vi "Battery Match.vi"(6 "ES ON Array In":bool[](array[boolean])=[FALSE, FALSE, FALSE, FALSE, FALSE, FALSE, FALSE, FALSE, FALSE, FALSE], 7 "Init":bool, 8 "Error In":errorcluster, 9 "PC Data":T2 {"Alarms 2" format="%016b"; "Faults 2" format="%016b"; "Alarms 1" format="%016b"; "Faults 1" format="%016b"; "Contactor FB" format="%.0b"; "DC Voltage SP" format="%2.1f"; "Clear Faults SP" format="%.0b"; "Neutral Current" format="%2.1f"; "AC Current - L2" format="%2.1f"; "AC Voltage - L2" format="%2.1f"; "Temperature" format="%2.1f"; "DC Voltage" format="%2.1f"; "AC Current SP" format="%2.1f"; "AC Voltage SP" format="%2.1f"; "Frequency SP" format="%2.1f"; "AC Frequency" format="%2.1f"; "AC Current - L1" format="%2.1f"; "AC Voltage- L1" format="%2.1f"}, 10 "ES System Data":T4={"Voltage"=0.0, "Current"=0.0, "SOC Avg"=0.0, "Faults"=0, "Alarms"=0, "# Strings"=0, "Max Temp"=0, "Min Temp"=0, "Max Cell Voltage"=0.0, "Min Cell Voltage"=0.0, "Energy Capacity"=0.0, "Energy Remaining"=0.0, "SOC Min"=0.0, "SOC Max"=0.0, "ES Fault"=FALSE, "String Select"=enum."3 Strings", "ES Com Fault"=FALSE, "SOH Avg"=0.0}, 11 "ES String Data":T6) -> (0 "Error Out":errorcluster, 1 "Matching Complete":bool=TRUE, 2 "ES ON Array Out":bool[](array[boolean]), 3 "Precharge Current Out":sgl)   [LabVIEW 2014]
uses:
  Controls/ES String Array.ctl
  Controls/ES String Data.ctl
  Controls/ES System Data.ctl
  Controls/StringSelector.ctl
  Controls/PC Data.ctl
  Controls/MicroZed Config Op Mode.ctl
  Controls/Battery Match State.ctl
panel:
  out "Last State":T1
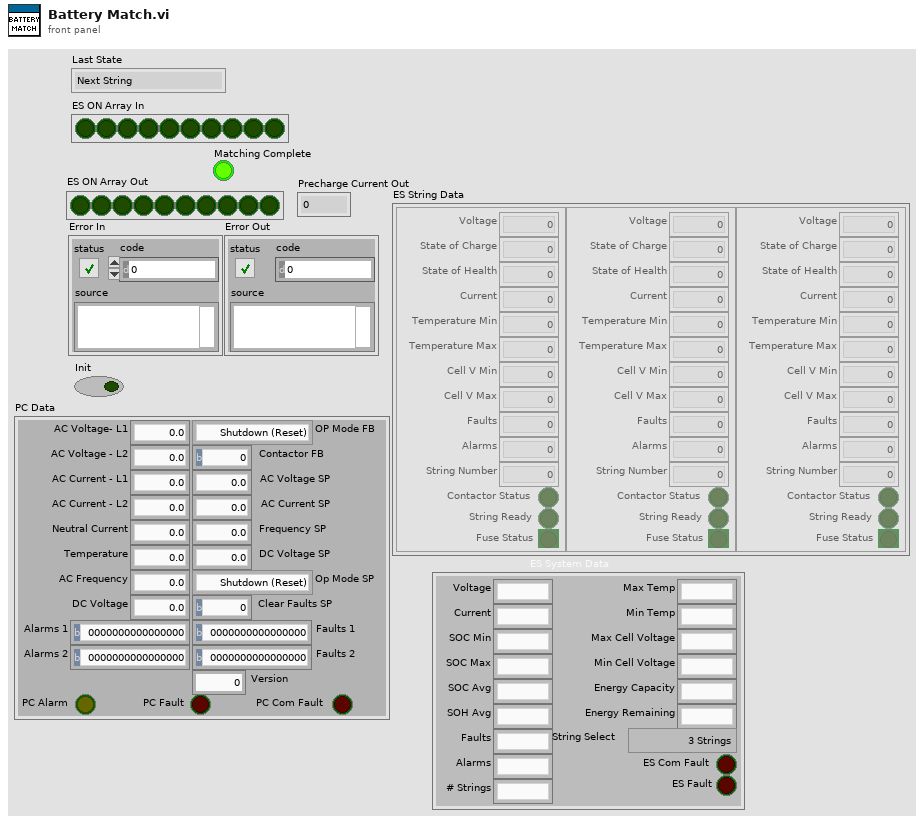
[diagram p1: front panel]
types:
  T1 = typedef "Battery Match State.ctl" = enum16{"Next String", "Charge String", "Matching Complete"}
  T2 = typedef "PC Data.ctl" = cluster{"AC Voltage- L1":dbl, "AC Voltage - L2":dbl, "AC Current - L1":dbl, "AC Current - L2":dbl, "Neutral Current":dbl, "Temperature":dbl, "AC Frequency":dbl, "DC Voltage":dbl, "AC Voltage SP":dbl, "AC Current SP":dbl, "Frequency SP":dbl, "Op Mode SP":T3, "Clear Faults SP":u16, "PC Com Fault":bool, "PC Fault":bool, "DC Voltage SP":dbl, "OP Mode FB":T3, "Contactor FB":u16, "Faults 1":u16, "Alarms 1":u16, "Faults 2":u16, "Alarms 2":u16, "PC Alarm":bool, "Version":u16}
  T3 = typedef "MicroZed Config Op Mode.ctl" = enum16{"Shutdown (Reset)", "Startup", "Idle", "Voltage Mode", "Current Mode", "Fault", "OL Voltage (Debug)", "No Data"}
  T4 = typedef "ES System Data.ctl" = cluster{"Voltage":sgl, "Current":sgl, "SOC Avg":sgl, "Faults":u16, "Alarms":u16, "# Strings":u16, "Max Temp":i16, "Min Temp":i16, "Max Cell Voltage":sgl, "Min Cell Voltage":sgl, "Energy Capacity":sgl, "Energy Remaining":sgl, "SOC Min":sgl, "SOC Max":sgl, "ES Fault":bool, "String Select":T5, "ES Com Fault":bool, "SOH Avg":sgl}
  T5 = typedef "StringSelector.ctl" = enum16{"1 String (1)", "1 String (2)", "1 String (3)", "2 Strings (1 2)", "2 Strings (2 3)", "2 Strings (1 3)", "3 Strings"}
  T6 = typedef "ES String Array.ctl" = T7[]
  T7 = typedef "ES String Data.ctl" = cluster{"Voltage":sgl, "State of Charge":sgl, "Current":sgl, "Temperature Min":i16, "Temperature Max":i16, "Faults":u16, "Alarms":u16, "String Number":u16, "Contactor Status":bool, "String Ready":bool, "Fuse Status":bool, "Cell V Max":dbl, "Cell V Min":dbl, "State of Health":sgl}
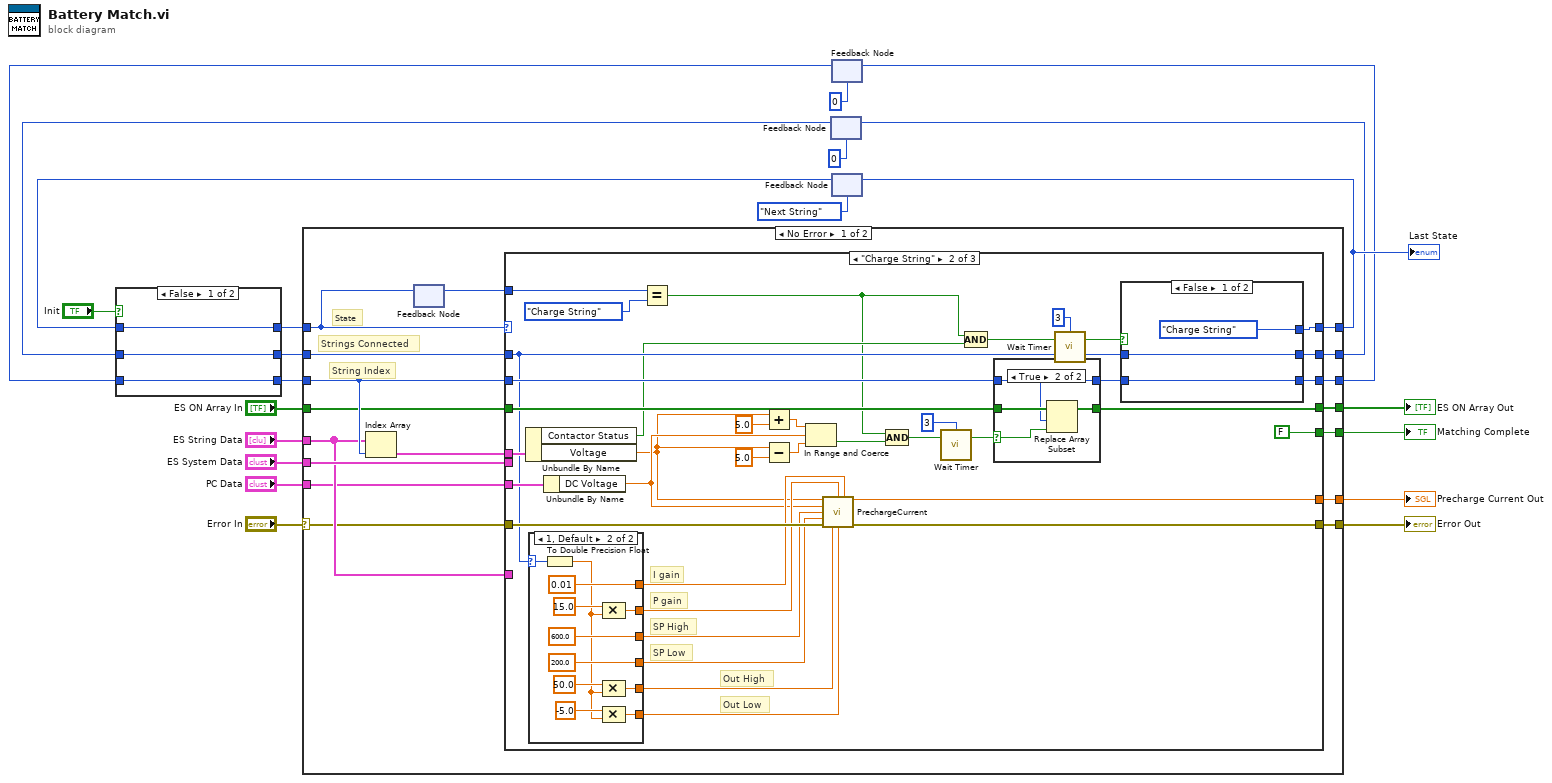
[diagram p0: block diagram]
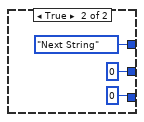
[diagram p2: hidden frame]
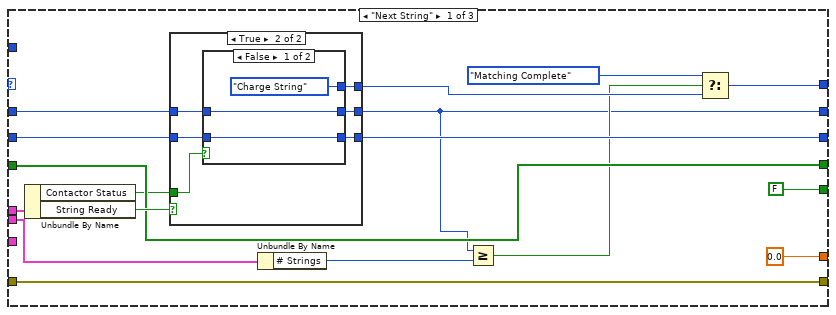
[diagram p3: hidden frame]
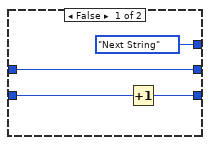
[diagram p4: hidden frame]
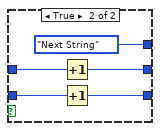
[diagram p5: hidden frame]
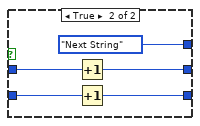
[diagram p6: hidden frame]
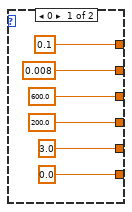
[diagram p8: hidden frame]
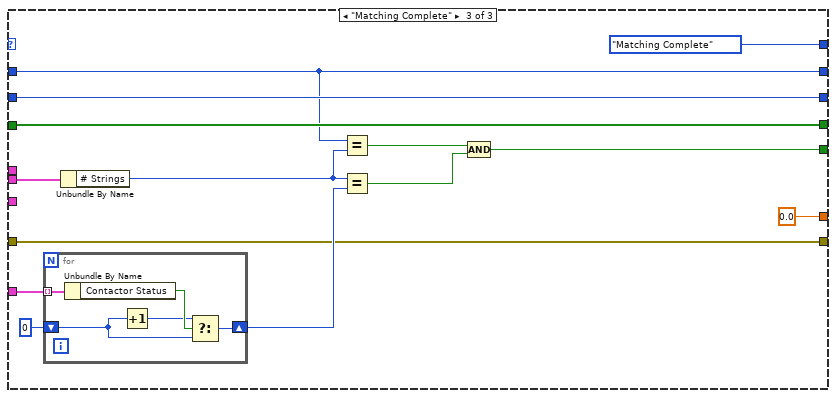
[diagram p9: hidden frame]
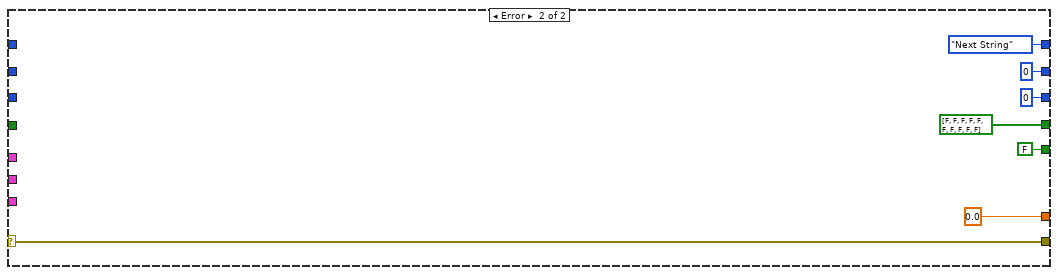
[diagram p10: hidden frame]
diagram:
  n1 = feedback #1(u16 0 ("index")) -> (w4:u16)
  n2 = feedback #2(0 ("index")) -> (w6:i32)
  n3 = feedback #3(Battery_Match_State."Next String") -> (w2:T1)
  n4 = case shown="False" "Init" {
    tunnel: w6 -> [w23 _]
    tunnel: w4 -> [w24 _]
    tunnel: w2 -> [w25 _]
    tunnel: [w25 Battery_Match_State."Next String"] -> w1
    tunnel: [w24 u16 0 ("index")] -> w3
    tunnel: [w23 0 ("index")] -> w5
    frame False {
    }
    frame True {
    }
  }
  n5 = case shown="No Error" "Error In" {
    selector: "Error In" -> [w32 w174]
    tunnel: [w33 w174] -> w21
    tunnel: "ES String Data" -> [w34 _]
    tunnel: "ES System Data" -> [w45 _]
    tunnel: "PC Data" -> [w31 _]
    tunnel: w5 -> [w42 _]
    tunnel: w1 -> [w30 _]
    tunnel: [w43 Battery_Match_State."Next String"] -> w15
    tunnel: [w41 0 ("index")] -> w14
    tunnel: "ES ON Array In" -> [w40 _]
    tunnel: [w39 bool[] [FALSE, FALSE, FALSE, FALSE, FALSE, FALSE, FALSE, FALSE, FALSE, FALSE] ("ES ON Array")] -> w13
    tunnel: w3 -> [w38 _]
    tunnel: [w37 FALSE] -> w11
    tunnel: [w36 sgl 0.0 ("Precharge Current Out")] -> w10
    tunnel: [w35 u16 0 ("index")] -> w9
    frame No Error {
      # "State"
      # "Strings Connected"
      # "String Index"
      n6 = Index Array(array=w34, index=w42) -> (element=w44:T7)
      n7 = feedback #4() -> (w29:T1)  [unwired: 1 in]
      n8 = feedback-in #4(w30) -> ()
      n9 = case shown="\"Charge String\"" w30 {
        tunnel: w45 -> [w52 _ w161]
        tunnel: w44 -> [w62 w108 _]
        tunnel: [w55 w92 Battery_Match_State."Matching Complete"] -> w43
        tunnel: w42 -> [w60 w104 w151]
        tunnel: [w58 w95 w151] -> w41
        tunnel: w40 -> [w59 w107 w153]
        tunnel: [w59 w106 w153] -> w39
        tunnel: w38 -> [w47 w94 w150]
        tunnel: [FALSE FALSE w152] -> w37
        tunnel: [sgl 0.0 ("Precharge Current Out") w117 sgl 0.0 ("Precharge Current Out")] -> w36
        tunnel: [w46 w93 w150] -> w35
        tunnel: w34 -> [_ _ w160]
        tunnel: [w56 w116 w154] -> w33
        tunnel: w32 -> [w56 w115 w154]
        tunnel: w31 -> [_ w105 _]
        tunnel: w29 -> [_ w83 _]
        frame "Next String" {
          n10 = Unbundle By Name(w62) -> ("Contactor Status"=w48:bool, "String Ready"=w61:bool)
          n11 = case shown="True" w61 {
            tunnel: [Battery_Match_State."Next String" w72] -> w54
            tunnel: w60 -> [w65 w68]
            tunnel: [w64 w67] -> w58
            tunnel: w48 -> [_ w71]
            tunnel: w47 -> [w63 w70]
            tunnel: [w63 w69] -> w46
            frame False {
              n12 = Increment(x=w65) -> (x+1=w64:i32)
            }
            frame True {
              n13 = case shown="False" w71 {
                tunnel: [Battery_Match_State."Charge String" Battery_Match_State."Next String"] -> w72
                tunnel: w70 -> [w75 w79]
                tunnel: [w75 w78] -> w69
                tunnel: w68 -> [w73 w77]
                tunnel: [w73 w76] -> w67
                frame False {
                }
                frame True {
                  n14 = Increment(x=w79) -> (x+1=w78:u16)
                  n15 = Increment(x=w77) -> (x+1=w76:i32)
                }
              }
            }
          }
          n16 = Unbundle By Name(w52) -> ("# Strings"=w51:u16)
          n17 = Greater Or Equal?(x=w46, y=w51) -> (x >= y?=w50:bool)
          n18 = Select(t=Battery_Match_State."Matching Complete", s=w50, f=w54) -> (s? t:f=w55:T1)
        }
        frame "Charge String" {
          # "Out Low"
          # "Out High"
          # "SP Low"
          # "SP High"
          # "P gain"
          # "I gain"
          n19 = Unbundle By Name(w108) -> ("Contactor Status"=w85:bool, "Voltage"=w90:sgl)
          n20 = case shown="1, Default" w94 {
            selector: w94 -> [_ w139]
            tunnel: [0.1 ("GainI") 0.01 ("GainI")] -> w114
            tunnel: [0.008 ("GainP") w142] -> w113
            tunnel: [3.0 ("Output High") w141] -> w110
            tunnel: [0.0 ("Output Low") w140] -> w109
            tunnel: [200.0 ("Setpoint Low") 200.0 ("Setpoint Low")] -> w111
            tunnel: [600.0 ("Setpoint High") 600.0 ("Setpoint High")] -> w112
            frame 0 {
            }
            frame 1, Default {
              n21 = To Double Precision Float(number=w139) -> (double precision float=w138:dbl)
              n22 = Compound Arithmetic op=MULTIPLY(15.0 ("GainP"), w138) -> (w142:dbl)
              n23 = Compound Arithmetic op=MULTIPLY(50.0 ("Output High"), w138) -> (w141:dbl)
              n24 = Compound Arithmetic op=MULTIPLY(-5.0 ("Output Low"), w138) -> (w140:dbl)
            }
          }
          n25 = Unbundle By Name(w105) -> ("DC Voltage"=w102:dbl)
          n26 = Equal?(x=w83, y=Battery_Match_State."Charge String") -> (x = y?=w81:bool)
          n27 = Add(x=w90, y=sgl 5.0) -> (x+y=w101:sgl)
          n28 = Subtract(x=w90, y=sgl 5.0) -> (x-y=w100:sgl)
          n29 = In Range and Coerce(upper limit=w101, x=w102, lower limit=w100) -> (In Range?=w86:bool)  [unwired: 1 out]
          n30 = call "PrechargeCurrent.vi"("Storage Voltage In (SP)"=w90, "GainP"=w113, "GainI"=w114, "Drive Voltage In (PV)"=w102, "Setpoint High"=w112, "Setpoint Low"=w111, "Error In"=w115, "Output High"=w110, "Output Low"=w109) -> ("Precharge Current Out"=w117:sgl, "Error Out"=w116:errorcluster)  [unwired: 5 in]
          n31 = Compound Arithmetic op=AND(w81, w86) -> (w87:bool)
          n32 = call "Wait Timer.vi"("Boolean In"=w87, "Timer"=u32 3) -> ("Boolean Out"=w98:bool)  [unwired: 3 in]
          n33 = Compound Arithmetic op=AND(w81, w85) -> (w84:bool)
          n34 = case shown="True" w98 {
            selector: w98 -> [_ w129]
            tunnel: w107 -> [w127 w131]
            tunnel: [w127 w130] -> w106
            tunnel: w104 -> [w126 w128]
            tunnel: [w126 w128] -> w96
            frame False {
            }
            frame True {
              n35 = Replace Array Subset(array=w131, new element=w129, index=w128) -> (w130:bool[])
            }
          }
          n36 = call "Wait Timer.vi"("Boolean In"=w84, "Timer"=u32 3) -> ("Boolean Out"=w91:bool)  [unwired: 3 in]
          n37 = case shown="False" w91 {
            tunnel: w96 -> [w120 w125]
            tunnel: [w120 w124] -> w95
            tunnel: w94 -> [w119 w123]
            tunnel: [w119 w122] -> w93
            tunnel: [Battery_Match_State."Charge String" Battery_Match_State."Next String"] -> w92
            frame False {
            }
            frame True {
              n38 = Increment(x=w123) -> (x+1=w122:u16)
              n39 = Increment(x=w125) -> (x+1=w124:i32)
            }
          }
        }
        frame "Matching Complete" {
          n40 = for {
            tunnel: w160 -> [w167] mode=indexing
            shift-right: [w163] -> w156
            shift-left: u16 0 -> [w165]
            n41 = Unbundle By Name(w167) -> ("Contactor Status"=w166:bool)
            n42 = Increment(x=w165) -> (x+1=w164:u16)
            n43 = Select(t=w164, s=w166, f=w165) -> (s? t:f=w163:u16)
          }
          n44 = Unbundle By Name(w161) -> ("# Strings"=w155:u16)
          n45 = Equal?(x=w150, y=w155) -> (x = y?=w158:bool)
          n46 = Equal?(x=w155, y=w156) -> (x = y?=w159:bool)
          n47 = Compound Arithmetic op=AND(w158, w159) -> (w152:bool)
        }
      }
    }
    frame Error {
    }
  }
  "Precharge Current Out" <- w10
  "ES ON Array Out" <- w13
  "Error Out" <- w21
  "Matching Complete" <- w11
  "Last State" <- w15
  n48 = feedback-in #1(w9) -> ()
  n49 = feedback-in #2(w14) -> ()
  n50 = feedback-in #3(w15) -> ()
